vi "Topo & GridSpectr_DriftCorrection_v5.vi"(6 "Internal use":string, 7 "Grid param":T2 {"height (m)" format="%#_6p"; "width (m)" format="%#_6p"; "center Y (m)" format="%#_6p"; "center X (m)" format="%#_6p"}, 8 "Error in (no error)":errorcluster, 9 "Points Y/Index Y":i32, 10 "Points X/Index X":i32, 11 "Method":enum16{"init", "run", "end"}(ring)=enum."end") -> (0 "Error out":errorcluster)   [LabVIEW 2014]
doc: "Example of a measurement VI to be used in the \"Experiments on a Grid\" tool as external VI.\n\nThis example measure the topography and spectroscopy data. The spectroscopy measurements are taken on a subgrid. The data are saved to a sxm and a binary file.\n\n- Nanonis Programming Interface -"
uses:
  <userlib>/Nanonis Prog Interface V5/Nanonis Prog Interface.lvlib
panel:
  in  "tip Speed (m/s)":sgl=1e-08 format="%.2p"
  in  "Drift Correction 2":T1
  out "X drift":i32
  out "Y drift":i32
  out "Queue Steps":i32=40
  in  "StepsBack":i32=40
  in  "Channel index (0-23)":u8=14
  in  "File name":string="single_mol_shortSTS"
  in  "STS Current":dbl=9.999999717180685e-10 format="%#_6p"
  in  "Imaging Current":dbl=5.00000006675716e-11 format="%#_6p"
  in  "zdrift \nDuration (s)":dbl
  in  "Correct z drift":bool
  out "Status":string="finishing"
  in  "Drift correction Pixels":i32=256 caption="Pixels for drift correction"
  out "Y Offset":dbl
  out "X Offset":dbl
  out "Points taken":dbl=14.0
  in  "Drift Correction every":i32=64
  in  "Y subgrid spacing":u16=1
  in  "X subgrid spacing":u16=1
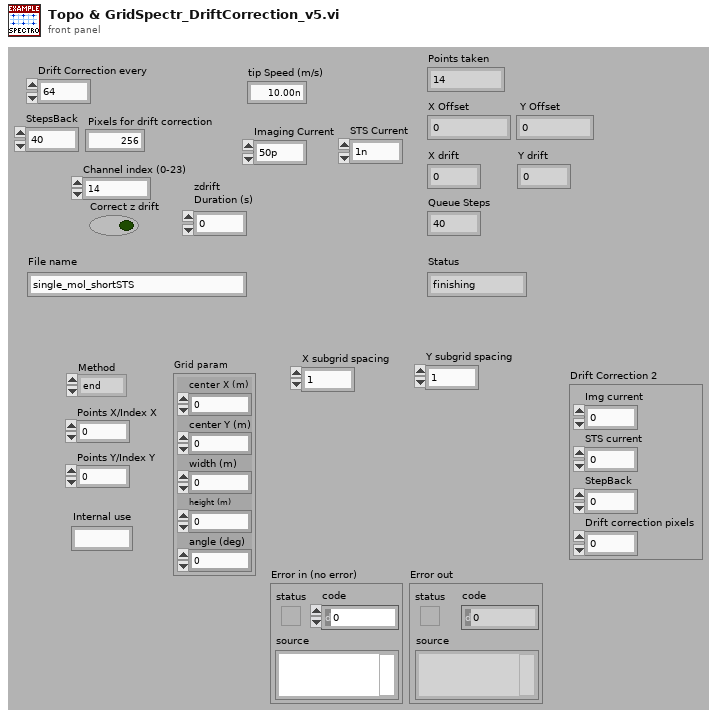
[diagram p1: front panel]
types:
  T1 = cluster{"Img current":dbl, "STS current":dbl, "StepBack":dbl, "Drift correction pixels":dbl}
  T2 = cluster{"center X (m)":sgl, "center Y (m)":sgl, "width (m)":sgl, "height (m)":sgl, "angle (deg)":sgl}
  T3 = cluster{"center X":sgl, "center Y":sgl, "angle":sgl, "width":sgl, "height":sgl, "# pixels":i32, "# lines":i32}
  T4 = cluster{"Name":string, "Calibration":sgl, "Offset":sgl, "Channel index":i32}[]
  T5 = cluster{"up/down":bool, "time/line":sgl, "start time":timestamp, "end time":timestamp}
  T6 = cluster{"Z averaging time (s)":sgl, "Z offset (m)":sgl, "Initial settling time (s)":sgl}
  T7 = cluster{"Max. slew rate (V/s)":sgl, "Settling time (s)":sgl, "Integration time (s)":sgl}
  T8 = cluster{"End settling time (s)":sgl, "Z control time (s)":sgl}
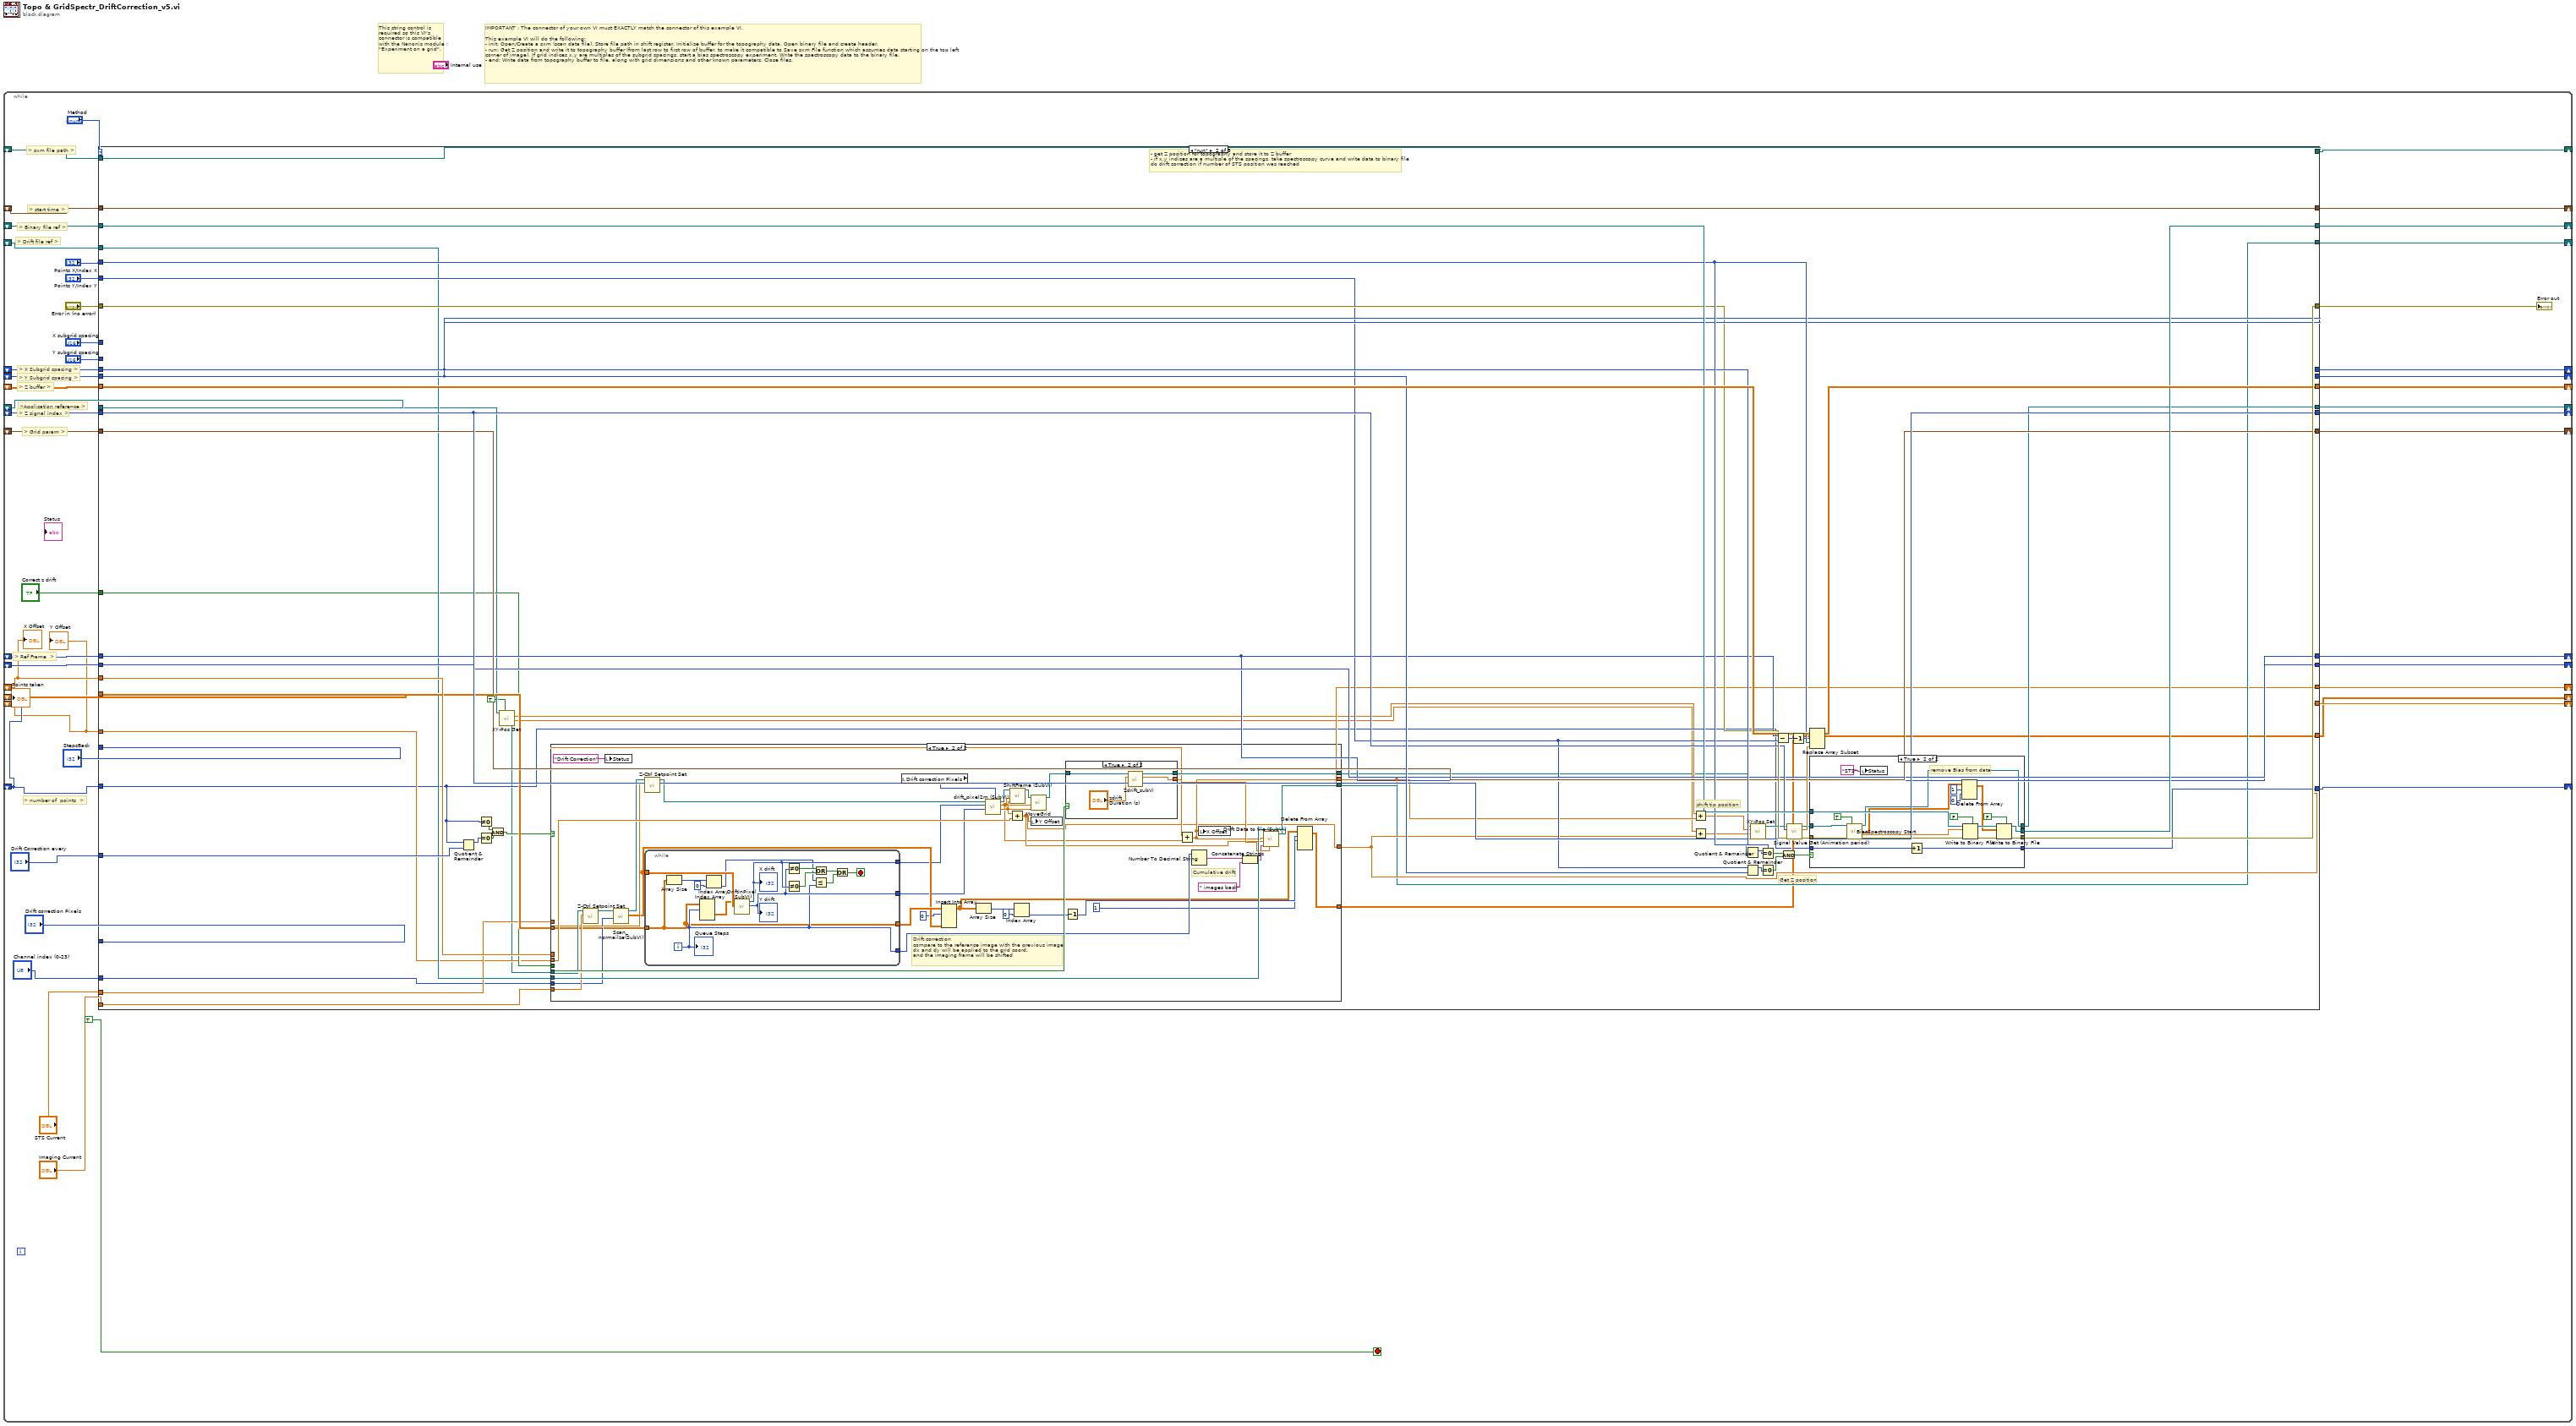
[diagram p0: block diagram]
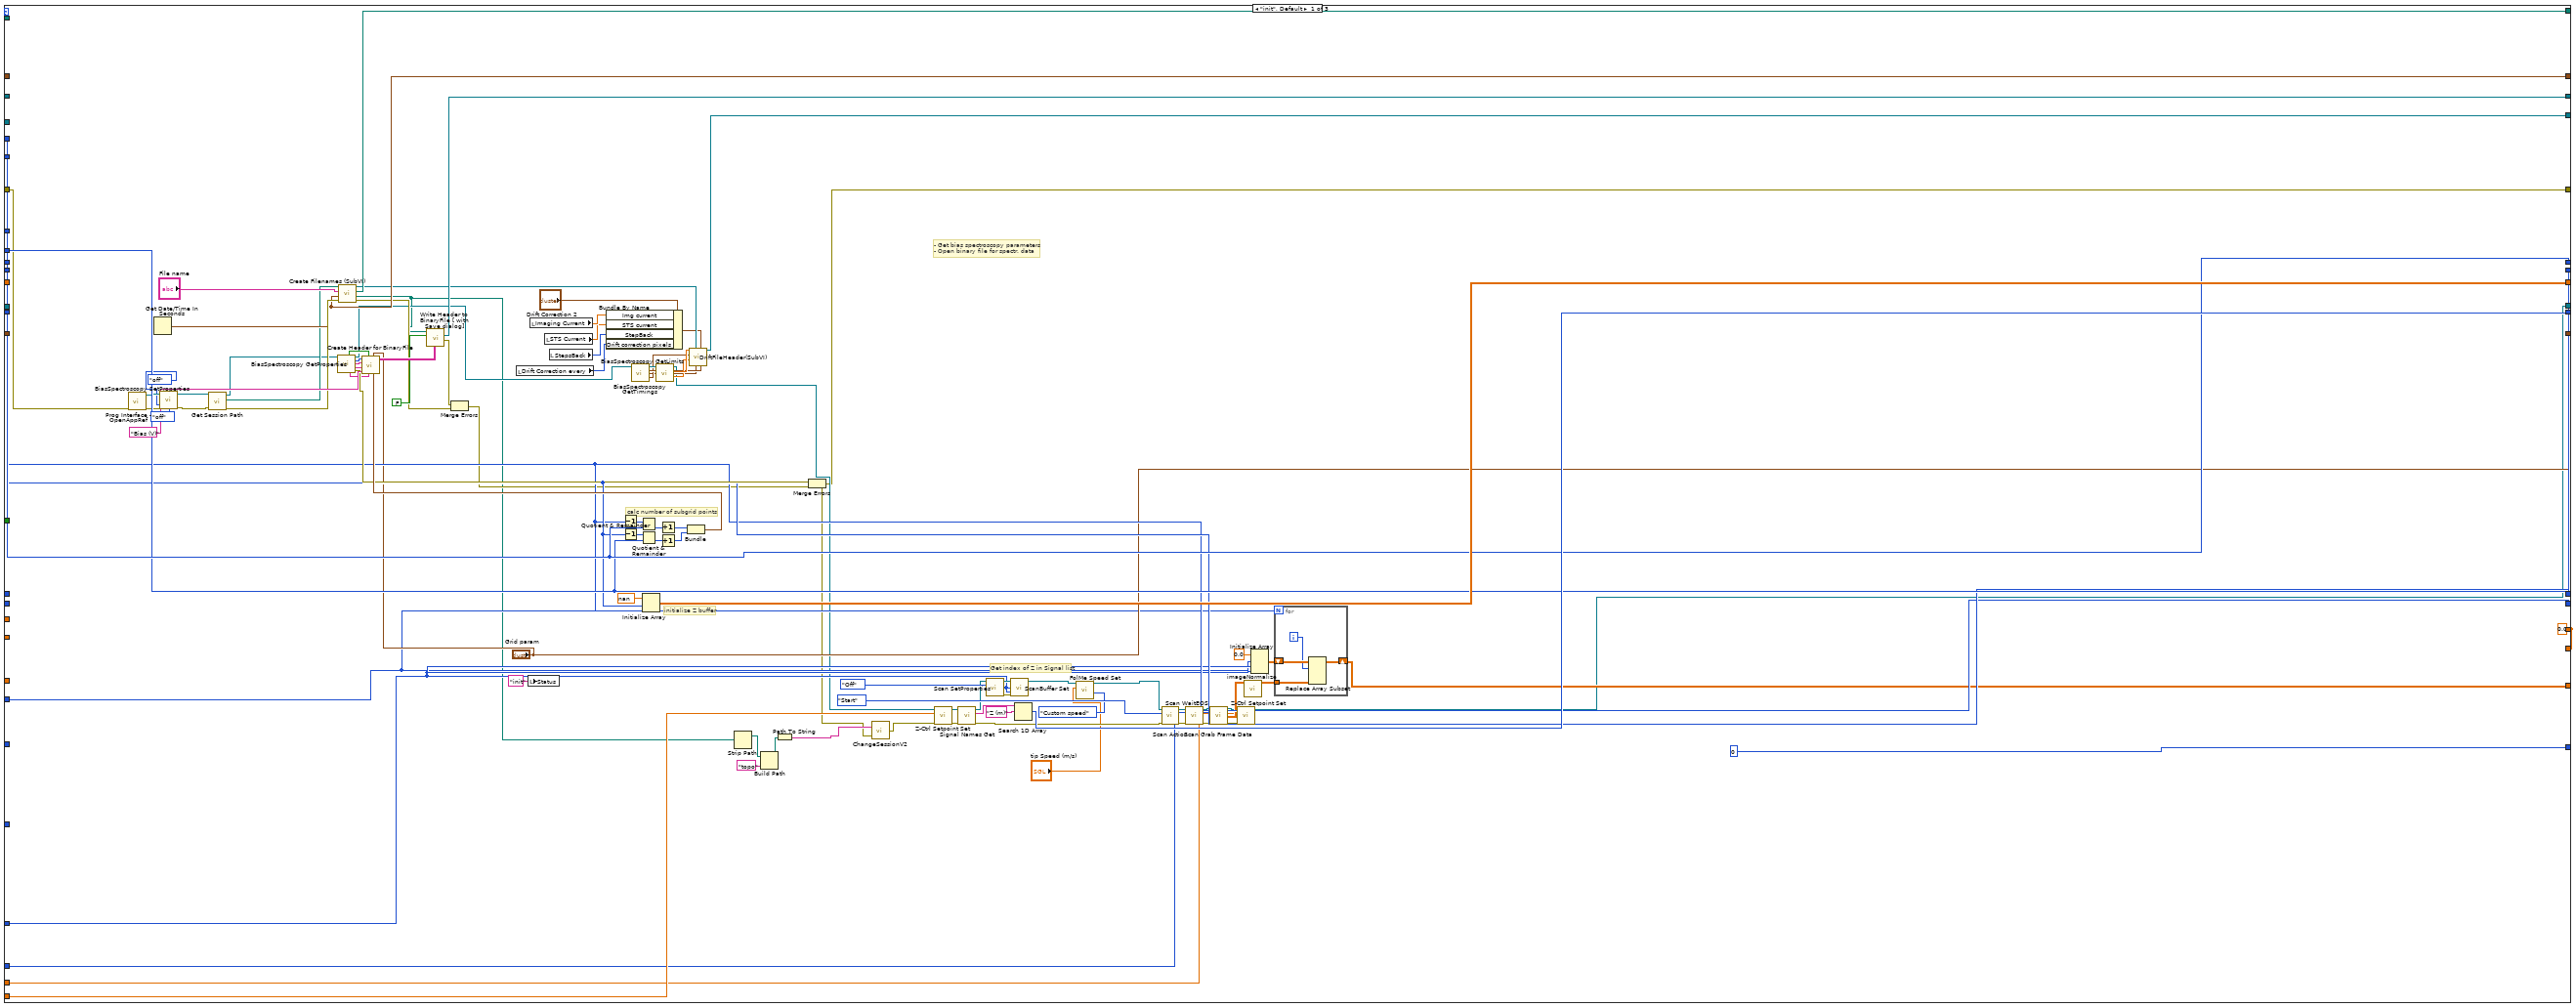
[diagram p2: hidden frame]
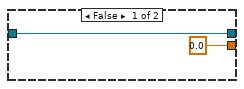
[diagram p4: hidden frame]
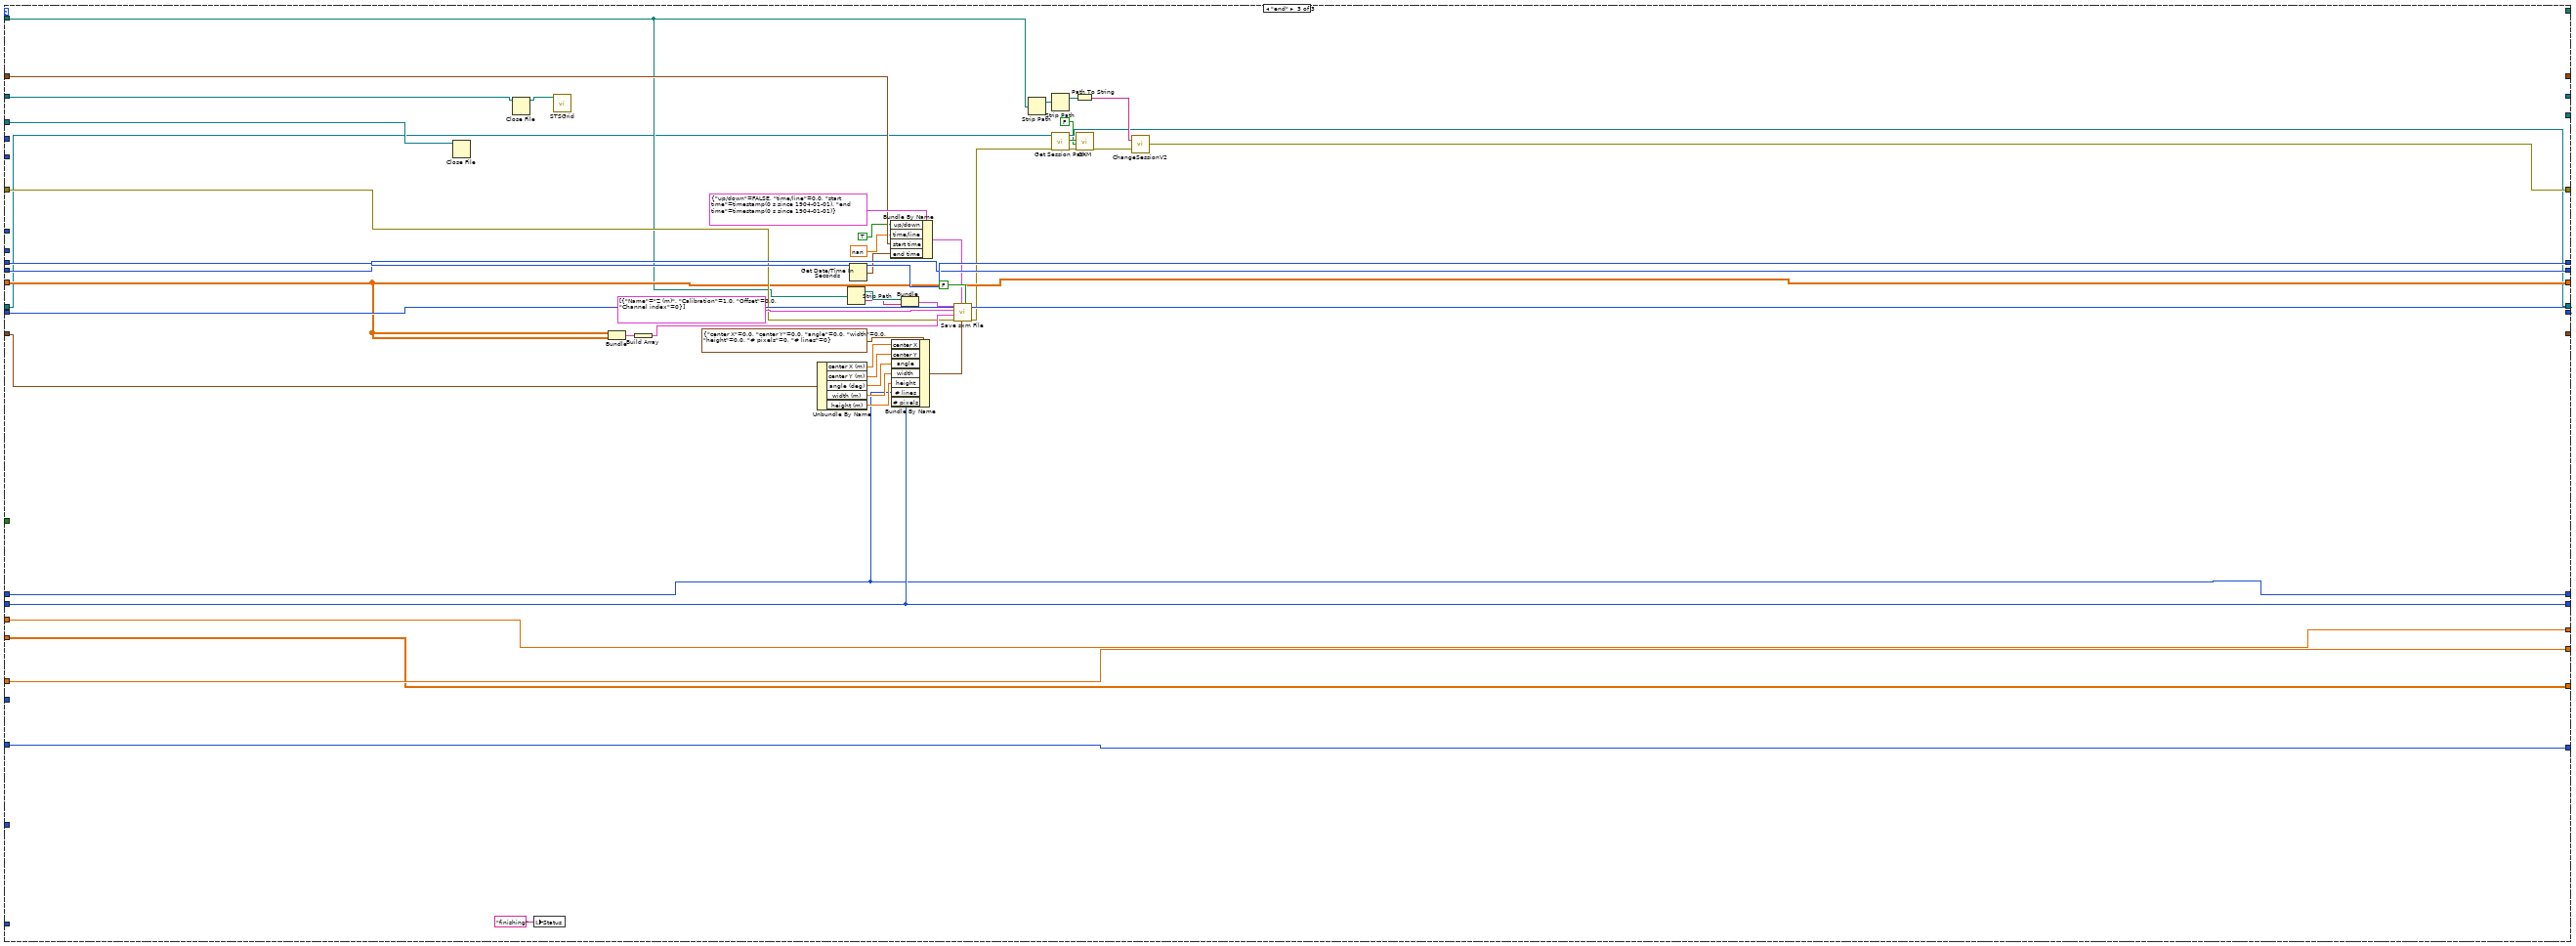
[diagram p6: hidden frame]
diagram:
  # "This string control is required so this VI's connector is compatible with the Nanonis module : \"Experiment on a grid\"."
  # "IMPORTANT : The connector of your own VI must EXACTLY match the connector of this example VI.\n\nThis example VI will do the following:\n- init: Open/Create a sxm (scan data file). Store file path in shift register. Initialize buffer for the topography data. Open binary file and create header.\n- run: Get Z position and write it to topography buffer (from last row to first row of buffer, to make it compatible to Save sxm File function which assumes data starting on the top left corner of image). If grid indices x,y are multiples of the subgrid spacings, start a bias spectroscopy experiment. Write the spectroscopy data to the binary file.\n- end: Write data from topography buffer to file, along with grid dimensions and other known parameters. Close files."
  n1 = while {
    shift-right: [w22] -> _
    shift-left: _ -> [w45]
    shift-right: [w40] -> _
    shift-left: _ -> [w39]
    shift-right: [w37] -> _
    shift-left: _ -> [w38]
    shift-right: [w36] -> _
    shift-left: _ -> [w35]
    shift-right: [w29] -> _
    shift-left: _ -> [w31]
    shift-right: [w30] -> _
    shift-left: _ -> [w32]
    shift-right: [w28] -> _
    shift-left: _ -> [w27]
    shift-right: [w26] -> _
    shift-left: _ -> [w25]
    shift-right: [w24] -> _
    shift-left: _ -> [w23]
    shift-right: [w21] -> _
    shift-left: _ -> [w20]
    shift-right: [w19] -> _
    shift-left: _ -> [w18]
    shift-right: [w17] -> _
    shift-left: _ -> [w10]
    shift-right: [w16] -> _
    shift-left: _ -> [w9]
    shift-right: [w15] -> _
    shift-left: _ -> [w12]
    shift-right: [w14] -> _
    shift-left: _ -> [w11]
    shift-right: [w7] -> _
    shift-left: _ -> [w6]
    stop <- TRUE stop-if-true
    # "> Drift file ref >"
    # "> number of  points  >"
    # "> Ref Frame  >"
    # "> Grid param >"
    # "> start time >"
    # ">Application reference >"
    # "> Y Subgrid spacing >"
    # "> X Subgrid spacing >"
    # "> Z signal index >"
    # "> Binary file ref >"
    # "> Z buffer >"
    # "> sxm file path >"
    n2 = case shown="\"run\"" "Method" {
      tunnel: [w95 w204 _] -> w22
      tunnel: w45 -> [_ w204 w304]
      tunnel: "Error in (no error)" -> [w97 w190 w327]
      tunnel: [w55 w203 w302] -> w43
      tunnel: "Points X/Index X" -> [w121 w198 _]
      tunnel: "Points Y/Index Y" -> [w122 w182 _]
      tunnel: [w145 w201 w316] -> w40
      tunnel: w39 -> [_ w202 w316]
      tunnel: w38 -> [_ w200 w308]
      tunnel: [w137 w199 _] -> w37
      tunnel: [w135 w188 w341] -> w36
      tunnel: w35 -> [_ w188 w341]
      tunnel: "X subgrid spacing" -> [w134 _ _]
      tunnel: "Y subgrid spacing" -> [w133 _ _]
      tunnel: w32 -> [_ w192 w340]
      tunnel: w31 -> [_ w191 w339]
      tunnel: [w134 w192 w340] -> w30
      tunnel: [w133 w191 w339] -> w29
      tunnel: [w68 w174 w298] -> w28
      tunnel: w27 -> [_ w155 w299]
      tunnel: ["Grid param" w185 _] -> w26
      tunnel: w25 -> [_ w185 w326]
      tunnel: [w94 w186 _] -> w24
      tunnel: w23 -> [_ w186 w334]
      tunnel: [w122 w183 w317] -> w21
      tunnel: w20 -> [_ w183 w317]
      tunnel: [w121 w184 w318] -> w19
      tunnel: w18 -> [_ w184 w318]
      tunnel: [w112 w164 w315] -> w17
      tunnel: [w112 w169 w313] -> w16
      tunnel: [w89 w161 w309] -> w15
      tunnel: [0 w179 w314] -> w14
      tunnel: w11 -> [_ w158 w314]
      tunnel: "Drift Correction every" -> [_ w177 _]
      tunnel: w12 -> [_ w168 w309]
      tunnel: w10 -> [_ w175 w315]
      tunnel: w9 -> [_ w159 w313]
      tunnel: "Drift correction Pixels" -> [w88 _ _]
      tunnel: [w84 w166 _] -> w7
      tunnel: w6 -> [_ w167 w310]
      tunnel: "Correct z drift" -> [_ w165 _]
      tunnel: "Imaging Current" -> [w103 w163 _]
      tunnel: "STS Current" -> [w99 w162 _]
      tunnel: "Channel index (0-23)" -> [w92 w160 _]
      tunnel: "StepsBack" -> [w87 _ _]
      frame "init", Default {
        w112 = 0.0
        # "- Get bias spectroscopy parameters\n- Open binary file for spectr. data"
        # "initialize Z buffer"
        # "calc number of subgrid points"
        # "Get index of Z in Signal list"
        n3 = call <userlib>:"Prog Interface - OpenAppRef.vi"("Error in (no error)"=w97) -> ("Error out"=w53:errorcluster, "Application reference"=w98:refnum<vi>)  [unwired: 5 in]
        n4 = Get Date/Time In Seconds() -> (seconds since 1Jan1904=w94:timestamp)
        n5 = call <userlib>:"BiasSpectroscopy SetProperties.vi"("Application ref in"=w98, "Autosave (no change)"=enum16{"no change", "on", "off"}."off", "Error in (no error)"=w53, "Save dialog"=enum16{"no change", "on", "off"}."off") -> ("Application ref out"=w49:refnum<vi>, "Error out"=w48:errorcluster)  [unwired: 10 in]
        n6 = call <userlib>:"Get Session Path.vi"("error in (no error)"=w48, "Application ref in"=w49) -> ("error out"=w96:errorcluster, "Session path"=w61:path, "Application ref out"=w50:refnum<vi>)  [unwired: 7 in]
        n7 = call <userlib>:"BiasSpectroscopy GetProperties.vi"("Application ref in"=w50) -> ("Backward sweep"=w141:bool, "Application ref out"=w67:refnum<vi>, "Number of points"=w124:i32, "Channels"=w123:string[], "Parameters"=w139:string[], "Fixed parameters"=w126:string[], "Error out"=w138:errorcluster)  [unwired: 6 in, 2 out]
        n8 = call "Create Filenames (SubVI).vi"("error in (no error)"=w96, "seconds since 1Jan1904"=w94, "File name"="File name", "Session path"=w61) -> ("error out"=w69:errorcluster, "binFilePath"=w57:path, "topoFilePath"=w95:path, "Drift File out"=w85:refnum<file>)  [unwired: 4 in]
        n9 = local read "Drift Correction every"() -> (w79:i32)
        n10 = local write "Status"("init" ("Status")) -> ()
        n11 = local read "Imaging Current"() -> (w81:dbl)
        n12 = local read "STS Current"() -> (w80:dbl)
        n13 = local read "StepsBack"() -> (w78:i32)
        n14 = Bundle By Name(cluster="Drift Correction 2", "Img current"=w81, "STS current"=w80, "StepBack"=w78, "Drift correction pixels"=w79) -> (w82:T1)
        n15 = Decrement(x=w121) -> (x-1=w132:i32)
        n16 = Decrement(x=w122) -> (x-1=w131:i32)
        n17 = call <userlib>:"BiasSpectroscopy GetTimings.vi"("Application ref in"=w67) -> ("Application ref out"=w77:refnum<vi>, "Initialization"=w74:T6, "Sweep Timing"=w72:T7, "End of Sweep"=w73:T8)  [unwired: 10 in, 1 out]
        n18 = Quotient & Remainder(x=w132, y=w134) -> (floor(x/y)=w130:i32)  [unwired: 1 out]
        n19 = Quotient & Remainder(x=w131, y=w133) -> (floor(x/y)=w129:i32)  [unwired: 1 out]
        n20 = Initialize Array(sgl nan ("element"), w122, w121) -> (w145:sgl[][])
        n21 = call <userlib>:"BiasSpectroscopy GetLimits.vi"("Application ref in"=w77) -> ("End value (V)"=w75:sgl, "Start value (V)"=w76:sgl, "Application ref out"=w66:refnum<vi>)  [unwired: 5 in, 1 out]
        n22 = Increment(x=w130) -> (x+1=w128:i32)
        n23 = Increment(x=w129) -> (x+1=w127:i32)
        n24 = Bundle(w128, w127) -> (w140:cluster{i32, i32})  [unwired: 1 in]
        n25 = call <userlib>:"Create Header for BinaryFile.vi"("Grid points"=w140, "Grid param"="Grid param", "Fixed parameters"=w126, "Backward sweep"=w141, "Sweep signal"="Bias (V)" ("Sweep Signal"), "Parameters"=w139, "Channels"=w123, "Points per sweep"=w124) -> ("Header (fixed attributes)"=w143:string[][])  [unwired: 3 in]
        n26 = call <userlib>:"Write Header to BinaryFile [ with Save dialog].vi"("Fixed Attributes"=w143, "Show Dialog? (T)"=FALSE, "Filename"=w57) -> ("Error out"=w70:errorcluster, "File ref"=w137:refnum<file>)  [unwired: 5 in, 2 out]
        n27 = Merge Errors(w70, w69) -> (w71:errorcluster)
        n28 = call "DriftFileHeader(SubVI).vi"("Initialization"=w74, "Drift Correction"=w82, "Sweep Timing"=w72, "Byte Stream File in"=w85, "End value (V)"=w75, "End of Sweep"=w73, "Start value (V)"=w76) -> ("Byte Stream File out"=w84:refnum<file>)  [unwired: 4 in]
        n29 = Strip Path(path=w57) -> (stripped path=w60:path)  [unwired: 1 out]
        n30 = Build Path(base path=w60, name or relative path="topo") -> (appended path=w58:path)
        n31 = Path To String(path=w58) -> (string=w56:string)
        n32 = Merge Errors(w138, w71) -> (w55:errorcluster)
        n33 = call "ChangeSessionV2.vi"("error in (no error)"=w55, "Session"=w56) -> ("error out"=w54:errorcluster)
        n34 = call <userlib>:"Z-Ctrl Setpoint Set.vi"("error in (no error)"=w54, "Z Controller setpoint"=w103, "Application ref in"=w66) -> ("error out"=w102:errorcluster, "Application ref out"=w104:refnum<vi>)  [unwired: 7 in]
        n35 = call <userlib>:"Signal Names Get.vi"("error in (no error)"=w102, "Application ref in"=w104) -> ("error out"=w113:errorcluster, "Signals Names"=w125:string[], "Application ref out"=w108:refnum<vi>)  [unwired: 5 in]
        n36 = call <userlib>:"Scan SetProperties.vi"("Application ref in"=w108, "Continuous scan"=enum16{"No change", "On", "Off"}."Off") -> ("Application ref out"=w110:refnum<vi>, "Error out"=w109:errorcluster)  [unwired: 12 in]
        n37 = call <userlib>:"ScanBuffer Set.vi"("Application ref in"=w110, "Pixels"=w88, "Lines"=w88, "error in (no error)"=w109) -> ("Application ref out"=w65:refnum<vi>)  [unwired: 10 in, 1 out]
        n38 = Search 1D Array(1D array=w125, element="Z (m)") -> (index of element=w135:i32)  [unwired: 1 in]
        n39 = call <userlib>:"FolMe Speed Set.vi"("Speed Setting (Custom)"=enum32{"Scan speed", "Custom speed"}."Custom speed", "Speed (m/s)"="tip Speed (m/s)", "Application ref in"=w65) -> ("Application ref out"=w64:refnum<vi>)  [unwired: 5 in, 1 out]
        n40 = call <userlib>:"Scan Action.vi"("error in (no error)"=w113, "Scan action (Start)"=enum16{"Start", "Stop", "Pause", "Resume"}."Start", "Application ref in"=w64) -> ("error out"=w119:errorcluster, "Application ref out"=w118:refnum<vi>)  [unwired: 6 in]
        n41 = call <userlib>:"Scan WaitEOS.vi"("error in (no error)"=w119, "Application ref in"=w118) -> ("error out"=w116:errorcluster, "Application ref out"=w117:refnum<vi>)  [unwired: 5 in, 2 out]
        n42 = call <userlib>:"Scan Grab Frame Data.vi"("Application ref in"=w117, "Channel index (0-23)"=w92, "error in (no error)"=w116) -> ("Application ref out"=w101:refnum<vi>, "Scan frame data"=w105:sgl[][], "error out"=w100:errorcluster)  [unwired: 8 in, 2 out]
        n43 = call <userlib>:"Z-Ctrl Setpoint Set.vi"("error in (no error)"=w100, "Z Controller setpoint"=w99, "Application ref in"=w101) -> ("Application ref out"=w68:refnum<vi>)  [unwired: 7 in, 1 out]
        n44 = call "imageNormalize.vi"("Data"=w105) -> ("Array"=w86:dbl[][])  [unwired: 10 in]
        n45 = Initialize Array(0.0 ("element"), w87, w88, w88) -> (w90:dbl[][][])
        n46 = for {
          N: w87 -> [_]
          tunnel: w86 -> [w148]
          shift-right: [w147] -> w89
          shift-left: w90 -> [w149]
          i -> [w146]
          n47 = Replace Array Subset(array=w149, new element=w148, index (dim 0)=w146) -> (w147:dbl[][][])  [unwired: 2 in]
        }
      }
      frame "run" {
        # "shift tip position"
        # "Get Z position"
        # "- get Z position for topography and store it to Z buffer\n- if x,y indices are a multiple of the spacings, take spectroscopy curve and write data to binary file\ndo drift correction if number of STS position was reached"
        n48 = Quotient & Remainder(x=w158, y=w177) -> (x-y*floor(x/y)=w178:i32)  [unwired: 1 out]
        n49 = Not Equal To 0?(x=w158) -> (x != 0?=w156:bool)
        n50 = Equal To 0?(x=w178) -> (x = 0?=w176:bool)
        n51 = And(x=w156, y=w176) -> (x .and. y?=w157:bool)
        n52 = call <userlib>:"XY-Pos Get.vi"("Wait for newest data (F=False)"=TRUE, "Application ref in"=w155) -> ("Y (m)"=w151:sgl, "X (m)"=w152:sgl, "Application ref out"=w154:refnum<vi>)  [unwired: 5 in, 1 out]
        n53 = case shown="True" w157 {
          tunnel: w154 -> [w209 w239]
          tunnel: [w209 w245] -> w150
          tunnel: w168 -> [w206 w233]
          tunnel: [w208 w241] -> w164
          tunnel: [w207 w240] -> w169
          tunnel: w175 -> [w208 w243]
          tunnel: w159 -> [w207 w244]
          tunnel: [w206 w225] -> w161
          tunnel: w167 -> [w205 w248]
          tunnel: [w205 w247] -> w166
          tunnel: w165 -> [_ w242]
          tunnel: w163 -> [_ w238]
          tunnel: w162 -> [_ w236]
          tunnel: w160 -> [_ w234]
          frame False {
          }
          frame True {
            # "Cumulative drift"
            # "Drift correction \ncompare to the reference image with the previous image \ndx and dy will be applied to the grid coord, \nand the imaging frame will be shifted"
            n54 = call <userlib>:"Z-Ctrl Setpoint Set.vi"("Z Controller setpoint"=w238, "Application ref in"=w239) -> ("Application ref out"=w235:refnum<vi>)  [unwired: 8 in, 1 out]
            n55 = local write "Status"("Drift Correction" ("Status")) -> ()
            n56 = call "Scan_normailze(SubVI).vi"("Channel index (0-23)"=w234, "Application in"=w235) -> ("Array"=w227:dbl[][], "Application out"=w237:refnum<vi>)  [unwired: 7 in, 1 out]
            n57 = call <userlib>:"Z-Ctrl Setpoint Set.vi"("Z Controller setpoint"=w236, "Application ref in"=w237) -> ("Application ref out"=w215:refnum<vi>)  [unwired: 8 in, 1 out]
            n58 = while {
              tunnel: w227 -> [w261]
              tunnel: w233 -> [w251]
              tunnel: [w260] -> w211
              tunnel: [w259] -> w210
              tunnel: [w255] -> w232
              tunnel: [w251] -> w228
              i -> [w255]
              stop <- w257 stop-if-true
              n59 = Array Size(array=w251) -> (size(s)=w254:i32[])
              n60 = Index Array(array=w251, index (dim 0)=w255) -> (element=w250:dbl[][])  [unwired: 2 in]
              n61 = Index Array(array=w254, index=0) -> (element=w252:i32)
              n62 = call "DriftInPixel (SubVI).vi"("New image"=w261, "Ref image"=w250) -> ("Y drift"=w259:i32, "X drift"=w260:i32)  [unwired: 7 in, 1 out]
              "Y drift" <- w259
              "X drift" <- w260
              n63 = Not Equal To 0?(x=w259) -> (x != 0?=w263:bool)
              n64 = Not Equal To 0?(x=w260) -> (x != 0?=w262:bool)
              n65 = Or(x=w263, y=w262) -> (x .or. y?=w258:bool)
              n66 = Less Or Equal?(x=w252, y=w255) -> (x <= y?=w256:bool)
              n67 = Or(x=w258, y=w256) -> (x .or. y?=w257:bool)
              "Queue Steps" <- w255
            }
            n68 = local read "Drift correction Pixels"() -> (w216:i32)
            n69 = Insert Into Array(array=w228, index (dim 0)=0 ("index (page)"), new element=w227) -> (w224:dbl[][][])  [unwired: 2 in]
            n70 = Array Size(array=w224) -> (size(s)=w223:i32[])
            n71 = call "drift_pixel2m (SubVI).vi"("Application in"=w215, "X drift"=w211, "Y drift"=w210, "Drift correction Pixels"=w216) -> ("Application out"=w214:refnum<vi>, "x drift"=w212:sgl, "y drift"=w213:sgl)  [unwired: 2 in, 1 out]
            n72 = Add(x=w213, y=w244) -> (x+y=w240:dbl)
            n73 = call "ShiftFrame (SubVI).vi"("Y shift"=w213, "X shift"=w212, "Application in"=w214) -> ("Application out"=w218:refnum<vi>)  [unwired: 8 in]
            n74 = Index Array(array=w223, index=0) -> (element=w221:i32)
            n75 = call "MoveGrid.vi"("y"=w213, "x"=w212, "Application ref in"=w218) -> ("Application ref out"=w217:refnum<vi>)  [unwired: 7 in, 1 out]
            n76 = local write "Y Offset"(w240) -> ()
            n77 = Decrement(x=w221) -> (x-1=w220:i32)
            n78 = case shown="True" w242 {
              tunnel: [0.0 ("z drift") w269] -> w246
              tunnel: w217 -> [w264 w268]
              tunnel: [w264 w267] -> w245
              frame False {
              }
              frame True {
                n79 = call "Zdrift_subVi.vi"("Duration"="zdrift \nDuration (s)", "Application in"=w268) -> ("z drift"=w269:dbl, "Application out"=w267:refnum<vi>)  [unwired: 7 in, 1 out]
              }
            }
            n80 = Add(x=w243, y=w212) -> (x+y=w241:dbl)
            n81 = Number To Decimal String(number=w232) -> (decimal integer string=w231:string)  [unwired: 1 in]
            n82 = local write "X Offset"(w241) -> ()
            n83 = Concatenate Strings(w231, " images back" ("string")) -> (w230:string)
            n84 = call "Drift Data to file (SubVI).vi"("z drift"=w246, "Comment"=w230, "y Drift"=w240, "X drift"=w241, "Byte Stream File in"=w248) -> ("Byte Stream File out"=w247:refnum<file>)  [unwired: 6 in]
            n85 = Delete From Array(array=w224, length=1, index (dim 0)=w220) -> (array with subset deleted=w225:dbl[][][])  [unwired: 2 in, 1 out]
          }
        }
        n86 = Add(x=w152, y=w164) -> (x+y=w171:dbl)
        n87 = Add(x=w151, y=w169) -> (x+y=w170:dbl)
        n88 = Quotient & Remainder(x=w198, y=w192) -> (x-y*floor(x/y)=w197:i32)  [unwired: 1 out]
        n89 = Quotient & Remainder(x=w182, y=w191) -> (x-y*floor(x/y)=w196:i32)  [unwired: 1 out]
        n90 = call <userlib>:"XY-Pos Set.vi"("Y (m)"=w170, "X (m)"=w171, "Application ref in"=w150) -> ("Application ref out"=w172:refnum<vi>)  [unwired: 5 in, 1 out]
        n91 = Equal To 0?(x=w197) -> (x = 0?=w195:bool)
        n92 = Equal To 0?(x=w196) -> (x = 0?=w194:bool)
        n93 = Subtract(x=w183, y=w182) -> (x-y=w181:i32)
        n94 = And(x=w195, y=w194) -> (x .and. y?=w193:bool)
        n95 = call <userlib>:"Signal Value Get (Animation period).vi"("error in (no error)"=w190, "Signal index (0-47)"=w188, "Application ref in"=w172) -> ("error out"=w189:errorcluster, "Signal value"=w187:sgl, "Application ref out"=w173:refnum<vi>)  [unwired: 5 in]
        n96 = Decrement(x=w181) -> (x-1=w180:i32)
        n97 = Replace Array Subset(array=w202, new element=w187, index (row)=w180, index (col)=w198) -> (w201:sgl[][])
        n98 = case shown="True" w193 {
          tunnel: [w272 w277] -> w203
          tunnel: w200 -> [w273 w293]
          tunnel: [w273 w291] -> w199
          tunnel: w189 -> [w272 w290]
          tunnel: w173 -> [w271 w282]
          tunnel: [w271 w281] -> w174
          tunnel: [w270 w275] -> w179
          tunnel: w158 -> [w270 w276]
          frame False {
            # "Point indices aren't multiple of subgrid spacing\n=> no spectroscopy at this point"
          }
          frame True {
            # "remove Bias from data"
            n99 = call <userlib>:"BiasSpectroscopy Start.vi"("Application ref in"=w282, "Get data (F)"=TRUE ("Get Data (F)"), "Error in (no error)"=w290) -> ("Application ref out"=w281:refnum<vi>, "Data"=w289:sgl[][], "Parameters"=w288:sgl[], "Error out"=w279:errorcluster)  [unwired: 8 in, 1 out]
            n100 = local write "Status"("STS" ("Status")) -> ()
            n101 = Increment(x=w276) -> (x+1=w275:i32)
            n102 = Delete From Array(array=w289, length=1, index (row)=0 ("index")) -> (array with subset deleted=w287:sgl[][])  [unwired: 1 in, 1 out]
            n103 = Write to Binary File(file (use dialog)=w293, data=w288, error in=w279, 5:FALSE ("prepend array or string size? (T)")) -> (refnum out=w292:refnum<file>, error out=w278:errorcluster)  [unwired: 2 in, 1 out]
            n104 = Write to Binary File(file (use dialog)=w292, data=w287, error in=w278, 5:FALSE ("prepend array or string size? (T)")) -> (refnum out=w291:refnum<file>, error out=w277:errorcluster)  [unwired: 2 in, 1 out]
          }
        }
      }
      frame "end" {
        n105 = Close File(refnum=w310) -> ()  [unwired: 1 in, 2 out]
        n106 = Close File(refnum=w308) -> (path=w307:path)  [unwired: 1 in, 1 out]
        n107 = local write "Status"("finishing" ("Status")) -> ()
        n108 = call "STSGrid.vi"("Binary Spectroscopy File"=w307) -> ()  [unwired: 11 in]
        n109 = Bundle(w316, w316) -> (w338:cluster{sgl[][], sgl[][]})  [unwired: 1 in]
        n110 = Build Array(w338) -> (w337:cluster{sgl[][], sgl[][]}[])
        n111 = Unbundle By Name(w326) -> ("center X (m)"=w324:sgl, "center Y (m)"=w323:sgl, "angle (deg)"=w322:sgl, "width (m)"=w321:sgl, "height (m)"=w320:sgl)
        n112 = Strip Path(path=w304) -> (stripped path=w330:path, name=w329:string)
        n113 = Get Date/Time In Seconds() -> (seconds since 1Jan1904=w312:timestamp)
        n114 = Bundle By Name(cluster=T5 {"up/down"=FALSE, "time/line"=0.0, "start time"=timestamp(0 s since 1904-01-01), "end time"=timestamp(0 s since 1904-01-01)} ("Scan param"), "up/down"=TRUE, "time/line"=sgl nan ("input 7"), "start time"=w334, "end time"=w312) -> (w333:T5)
        n115 = Bundle By Name(cluster=T3 {"center X"=0.0, "center Y"=0.0, "angle"=0.0, "width"=0.0, "height"=0.0, "# pixels"=0, "# lines"=0} ("Scanfield"), "center X"=w324, "center Y"=w323, "angle"=w322, "width"=w321, "height"=w320, "# lines"=w317, "# pixels"=w318) -> (w319:T3)
        n116 = Bundle("stripped path"=w330, "name"=w329) -> (w328:cluster{"stripped path":path, "name":string})  [unwired: 1 in]
        n117 = call <userlib>:"Save sxm File.vi"("Auto file naming? (T)"=FALSE, "Scanfield"=w319, "Scan param"=w333, "error in (no error)"=w327, "Channels data"=w337, "Channels config"=T4 [{"Name"="Z (m)", "Calibration"=1.0, "Offset"=0.0, "Channel index"=0}], "Filename control"=w328) -> ("error out"=w300:errorcluster)  [unwired: 2 in, 2 out]
        n118 = Strip Path(path=w304) -> (stripped path=w306:path)  [unwired: 1 out]
        n119 = Strip Path(path=w306) -> (stripped path=w305:path)  [unwired: 1 out]
        n120 = call <userlib>:"Get Session Path.vi"("error in (no error)"=w300, "Application ref in"=w299) -> ("error out"=w295:errorcluster, "Session path"=w297:path, "Application ref out"=w298:refnum<vi>)  [unwired: 7 in]
        n121 = Path To String(path=w305) -> (string=w301:string)
        n122 = call "SXM.vi"("Path"=w297, "Delete"=FALSE, "error in"=w295) -> ("error out"=w294:errorcluster)  [unwired: 7 in]
        n123 = call "ChangeSessionV2.vi"("error in (no error)"=w294, "Session"=w301) -> ("error out"=w302:errorcluster)
      }
    }
    "Error out" <- w43
    "Points taken" <- w11
    "X Offset" <- w10
    "Y Offset" <- w9
  }
